vi "Dymin_v5.vi"() -> ()   [LabVIEW 2016]
doc: "This VI demonstrates how to use an external signal to control the execution rate of a while loop."
uses:
  <vilib>/Platform/TimedLoop/XDataNode/wakeup.ctl
  <vilib>/Platform/TimedLoop/XDataNode/XDNodeRunTimeDep.lvlib
  <vilib>/Platform/TimedLoop/XDataNode/nitl_modes.ctl
  <vilib>/Platform/TimedLoop/XDataNode/timing_clust.ctl
  <vilib>/Platform/TimedLoop/XDataNode/XDataNode.xnode
  <vilib>/eio/EIONode/EIONode.xnode
  <vilib>/rvi/eio/common/nirviEmuTemplateMethod_errors.vi
  <vilib>/rvi/DataTransferAndStorage/Container/XNode/niFpgaContainer.xnode
  <vilib>/rvi/FIFO/Fifo_Resource/niFpgaFifoEmulationRefIn.vi
panel:
  out "Index":i32
  out "Dymin Step":i32
  out "Counts":i32
  out "Last Index":i32
  out "Last Counts":i32
  in  "Time (#80MHz periods)":i32[](array[numeric])=[32, 32, 32, 32]
  in  "Threshold (counts)":i32[](array[numeric])=[0, 0, 0, 0]
  in  "AOM Volts (V)":i32[](array[numeric])=[0, 82, 164, 246]
  # "12 bit ADC volts"
  # ".1=82\n.2=164\n.3=246"
  # "16=200ns\n32=400ns"
  # "0 value means the step before it was the last step"
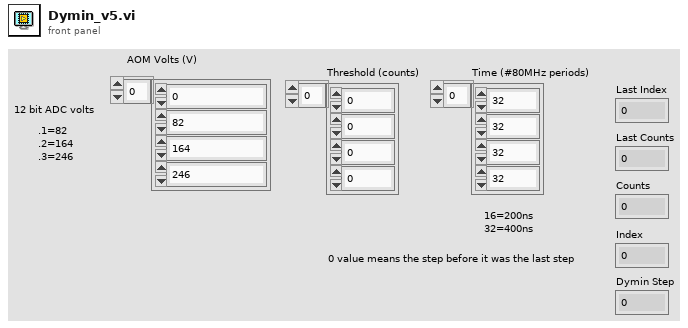
[diagram p1: front panel]
types:
  T1 = typedef "XDNodeRunTimeDep.lvlib/timing_clust.ctl" = cluster{"Expected End [f-1]":u64, "Actual End [f-1]":u64, "Finished Late? [f-1]":bool, "Expected End [i-1]":u64, "Actual End [i-1]":u64, "Finished Late? [i-1]":bool, "Expected Start [i]":u64, "Actual Start [i]":u64, "Expected Start [f]":u64, "Actual Start [f]":u64, "Source Name":string, "Structure Name":string, "Period":i64, "Deadline":i64, "Offset":i64, "Start":i64, "Priority":i32, "Timeout":i32, "Mode":T2, "Wakeup Reason":T3, "Error":errorcluster, "Source Type":string, "Secondary Source Type":string, "Global End Time":u64, "Global Start Time":u64, "Frame Duration":u64, "Iteration Duration":u64, "Assigned CPU":i32, "I/O Scan Engine Mode":u32}
  T2 = typedef "XDNodeRunTimeDep.lvlib/nitl_modes.ctl" = enum32{"No Change", "Process missed periods, maintain original phase", "Discard missed periods, maintain original phase", "Process missed periods, ignore original phase", "Discard missed periods, ignore original phase"}
  T3 = typedef "XDNodeRunTimeDep.lvlib/wakeup.ctl" = enum32{"Normal", "Aborted", "Asynchronous wakeup", "Timing source error", "Timed loop error", "Timeout"}
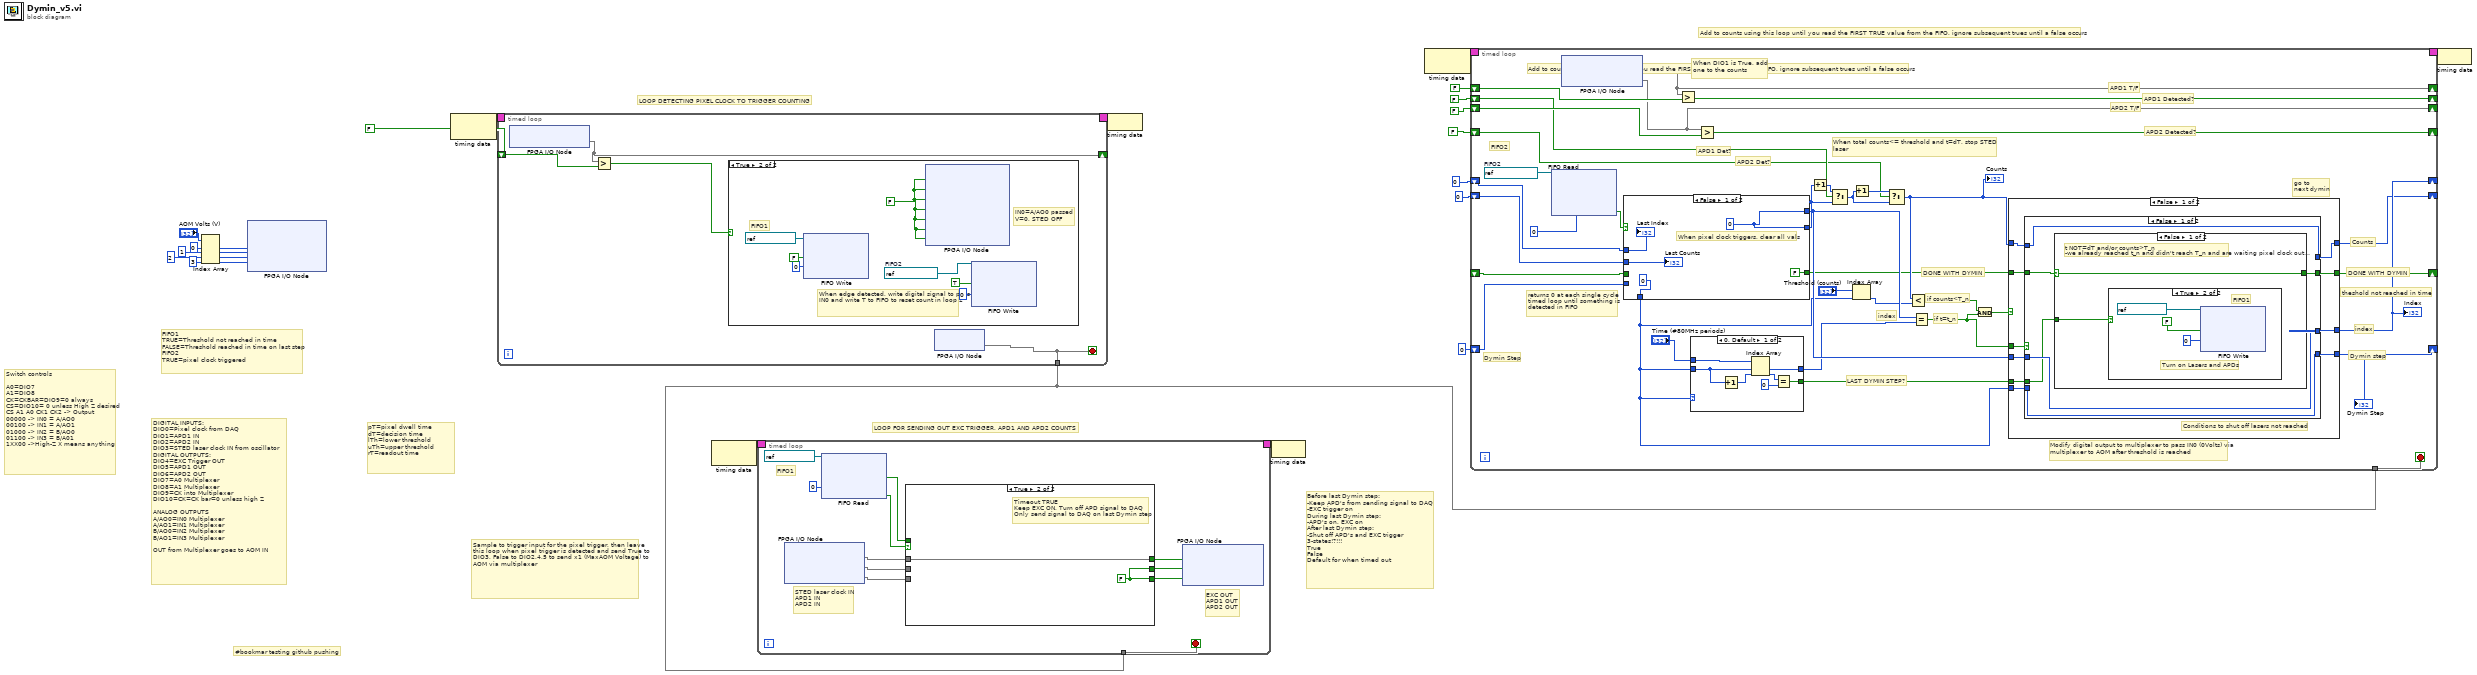
[diagram p0: block diagram]
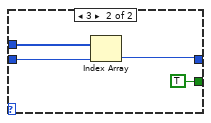
[diagram p2: hidden frame]
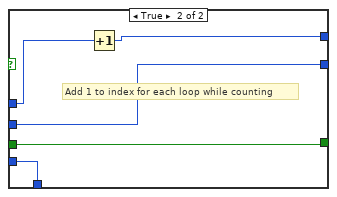
[diagram p3: hidden frame]
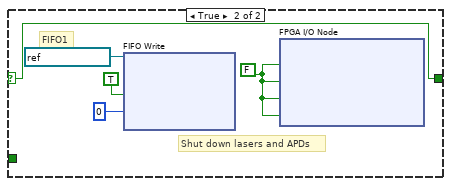
[diagram p5: hidden frame]
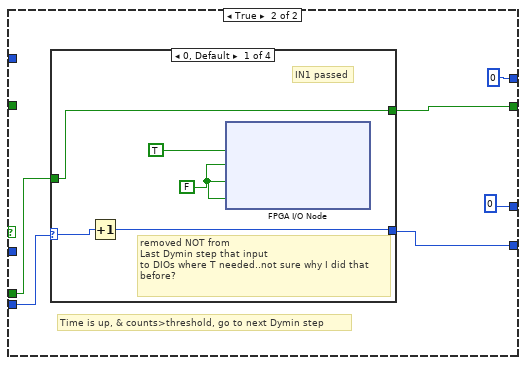
[diagram p6: hidden frame]
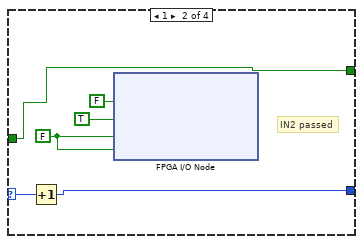
[diagram p7: hidden frame]
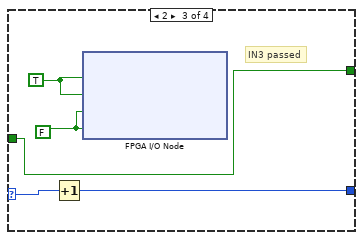
[diagram p8: hidden frame]
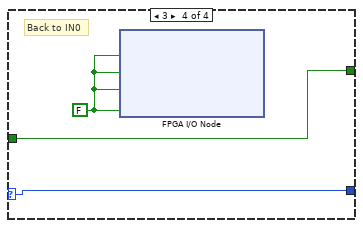
[diagram p9: hidden frame]
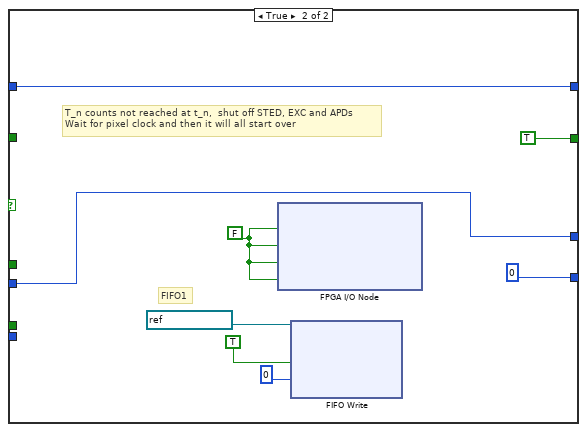
[diagram p10: hidden frame]
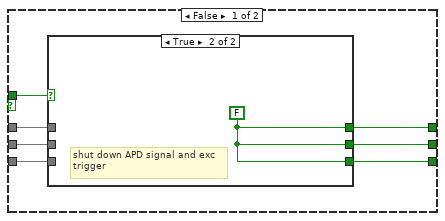
[diagram p11: hidden frame]
diagram:
  # "#bookmar testing github pushing"
  # "Switch controls\n\nA0=DIO7\nA1=DIO8\nCK=CKBAR=DIO9=0 always\nCS=DIO10= 0 unless High Z desired\nCS A1 A0 CK1 CK2 -> Output\n00000 -> IN0 = A/AO0\n00100 -> IN1 = A/AO1\n01000 -> IN2 = B/AO0\n01100 -> IN3 = B/A01\n1XX00 ->High-Z X means anything"
  # "FIFO1\nTRUE=Threshold not reached in time\nFALSE=Threshold reached in time on last step\nFIFO2\nTRUE=pixel clock triggered"
  # "DIGITAL INPUTS:\nDIO0=Pixel clock from DAQ\nDIO1=APD1 IN \nDIO2=APD2 IN\nDIO3=STED laser clock IN from oscillator\nDIGITAL OUTPUTS:\nDIO4=EXC Trigger OUT\nDIO5=APD1 OUT\nDIO6=APD2 OUT\nDIO7=A0 Multiplexer\nDIO8=A1 Multiplexer\nDIO9=CK into Multiplexer\nDIO10=CK=CK bar=0 unless high Z\n\nANALOG OUTPUTS\nA/AO0=IN0 Multiplexer\nA/AO1=IN1 Multiplexer\nB/AO0=IN2 Multiplexer\nB/AO1=IN3 Multiplexer\n\nOUT from Multiplexer goes to AOM IN"
  # "Before last Dymin step:\n-Keep APD's from sending signal to DAQ\n-EXC trigger on\nDuring last Dymin step:\n-APD's on, EXC on\nAfter last Dymin step:\n-Shut off APD's and EXC trigger\n3-states!?!!!\nTrue\nFalse\nDefault for when timed out"
  # "Add to counts using this loop until you read the FIRST TRUE value from the FIFO, ignore subsequent trues until a false occurs"
  # "LOOP FOR SENDING OUT EXC TRIGGER, APD1 AND APD2 COUNTS"
  # "LOOP DETECTING PIXEL CLOCK TO TRIGGER COUNTING"
  # "Add to counts using this loop until you read the FIRST TRUE value from the FIFO, ignore subsequent trues until a false occurs"
  # "Sample to trigger input for the pixel trigger, then leave this loop when pixel trigger is detected and send True to DIO3, False to DIO2,4,5 to send x1 (MaxAOM Voltage) to AOM via multiplexer"
  # "pT=pixel dwell time\ndT=decision time\nlTh=lower threshold\nuTh=upper threshold\nrT=readout time"
  n1 = Index Array(array="AOM Volts (V)", index #1=0 ("index"), index #2=1 ("index"), index #3=2 ("index"), index #4=3 ("index")) -> (element #1=w1:i32, element #2=w4:i32, element #3=w3:i32, element #4=w2:i32)
  n2 = xnode "FPGA I/O Node"("ConnectorA/AO0"=w1, "ConnectorA/AO1"=w4, "ConnectorB/AO0"=w3, "ConnectorB/AO1"=w2) -> ()  [unwired: 4 in, 4 out]
  n3 = node-c288() -> (w24:T1)  [unwired: 1 in]
  n4 = timed-loop {
    timing: w24 -> [_]
    timing-out: [_] -> w23
    shift-right: [w27] -> _
    shift-left: FALSE -> [w28]
    tunnel: [w25] -> w10
    stop <- w25 stop-if-true
    n5 = xnode "FPGA I/O Node"() -> ("ConnectorA/DIO0"=w27)  [unwired: 1 in, 1 out]
    n6 = Greater?(x=w27, y=w28) -> (0:w26:bool)
    n7 = case shown="True" w26 {
      frame False {
      }
      frame True {
        w29 = FALSE ("ConnectorA/DIO4")
        w35 = refnum<k21> "A.DO1 DMA"  # FIFO2
        # "FIFO1"
        # "When edge detected, write digital signal to pass IN0 and write T to FIFO to reset count in loop 2"
        # "IN0=A/AO0 passed\nV=0, STED OFF"
        n8 = xnode ("FIFO Write")("Element"=FALSE, "Timeout"=0, "FIFO In"=refnum<k21> "A.DI0 DMA") -> ()  [unwired: 2 out]
        n9 = xnode "FPGA I/O Node"("ConnectorA/DIO4"=w29, "ConnectorA/DIO5"=w29, "ConnectorA/DIO6"=w29, "ConnectorA/DIO7"=w29, "ConnectorA/DIO8"=w29, "ConnectorA/DIO9"=w29, "ConnectorA/DIO10"=w29) -> ()  [unwired: 7 in, 7 out]
        n10 = xnode ("FIFO Write")("Element"=TRUE, "Timeout"=0, "FIFO In"=w35) -> ()  [unwired: 2 out]
      }
    }
    n11 = xnode "FPGA I/O Node"() -> ("Button0"=w25)  [unwired: 1 in, 1 out]
  }
  n12 = node-c288() -> (w21:T1)  [unwired: 1 in]
  n13 = timed-loop {
    timing: w21 -> [_]
    timing-out: [_] -> w20
    tunnel: w10 -> [w38]
    stop <- w38 stop-if-true
    # "EXC OUT\nAPD1 OUT\nAPD2 OUT"
    # "FIFO1"
    # "STED laser clock IN\nAPD1 IN\nAPD2 IN"
    n14 = xnode "FPGA I/O Node"() -> ("ConnectorA/DIO3"=w46, "ConnectorA/DIO1"=w43, "ConnectorA/DIO2"=w42)  [unwired: 3 in, 3 out]
    n15 = xnode ("FIFO Read")("Timeout"=0, "FIFO In"=refnum<k21> "A.DI0 DMA") -> ("Element"=w45:bool, "Timed Out?"=w39:bool)  [unwired: 1 out]
    n16 = case shown="True" w39 {
      tunnel: w46 -> [w55 w61]
      tunnel: w45 -> [w54 _]
      tunnel: [w53 w61] -> w44
      tunnel: w43 -> [w52 _]
      tunnel: w42 -> [w51 _]
      tunnel: [w50 w60] -> w41
      tunnel: [w49 w60] -> w40
      frame False {
        n17 = case shown="True" w54 {
          tunnel: w55 -> [w58 _]
          tunnel: [w58 w59] -> w53
          tunnel: w52 -> [w57 _]
          tunnel: w51 -> [w56 _]
          tunnel: [w57 w59] -> w50
          tunnel: [w56 w59] -> w49
          frame False {
            # "Sends Exc Trig out, APD1 and APD2 out using FPGA"
          }
          frame True {
            w59 = FALSE ("ConnectorA/DIO3")
            # "shut down APD signal and exc trigger"
          }
        }
      }
      frame True {
        w60 = FALSE
        # "Timeout TRUE\nKeep EXC ON, Turn off APD signal to DAQ\nOnly send signal to DAQ on last Dymin step"
      }
    }
    n18 = xnode "FPGA I/O Node"("ConnectorA/DIO4"=w44, "ConnectorA/DIO5"=w41, "ConnectorA/DIO6"=w40) -> ()  [unwired: 3 in, 3 out]
  }
  n19 = node-c288(w23) -> ()
  n20 = node-c288(w20) -> ()
  n21 = node-c288() -> (w19:T1)  [unwired: 1 in]
  n22 = timed-loop {
    timing: w19 -> [_]
    timing-out: [_] -> w18
    shift-right: [w97] -> _
    shift-left: FALSE -> [w99]
    shift-right: [w91] -> _
    shift-left: FALSE -> [w86]
    shift-right: [w80] -> _
    shift-left: 0 -> [w94]
    shift-right: [w75] -> _
    shift-left: FALSE -> [w87]
    shift-right: [w92] -> _
    shift-left: FALSE -> [w90]
    shift-right: [w76] -> _
    shift-left: 0 -> [w88]
    shift-right: [w82] -> _
    shift-left: 0 -> [w66]
    shift-right: [w70] -> _
    shift-left: _ -> [w68]
    tunnel: w10 -> [w64]
    stop <- w64 stop-if-true
    w79 = refnum<k21> "A.DO1 DMA"  # FIFO2
    # "DONE WITH DYMIN"
    # "go to\nnext dymin"
    # "DONE WITH DYMIN"
    # "LAST DYMIN STEP?"
    # "theshold not reached in time"
    # "Dymin Step"
    # "Dymin step"
    # "FIFO2"
    # "if counts<T_n"
    # "if t=t_n"
    # "returns 0 at each single cycle timed loop until something is detected in FIFO"
    # "Modify digital output to multiplexer to pass IN0 (0Volts) via multiplexer to AOM after threshold is reached"
    # "When total counts<= threshold and t=dT, stop STED laser"
    # "index"
    # "APD1 Det?"
    # "APD2 Det?"
    # "APD2 Detected?"
    # "APD2 T/F"
    # "APD1 Detected?"
    # "APD1 T/F"
    # "index"
    # "Counts"
    # "When DIO1 is True, add one to the counts"
    n23 = xnode ("FIFO Read")("Timeout"=0, "FIFO In"=w79) -> ("Timed Out?"=w93:bool)  [unwired: 2 out]
    n24 = xnode "FPGA I/O Node"() -> ("ConnectorA/DIO1"=w97, "ConnectorA/DIO2"=w92)  [unwired: 2 in, 2 out]
    n25 = case shown="False" w93 {
      tunnel: [w114 w118] -> w95
      tunnel: [w114 w119] -> w81
      tunnel: w94 -> [w115 w120]
      tunnel: w88 -> [w113 w118]
      tunnel: w68 -> [_ w117]
      tunnel: [FALSE w117] -> w67
      tunnel: w66 -> [_ w116]
      tunnel: [0 w116] -> w65
      frame False {
        w114 = 0
        # "When pixel clock triggers, clear all vals"
        "Last Index" <- w115
        "Last Counts" <- w113
      }
      frame True {
        # "Add 1 to index for each loop while counting"
        n26 = Increment(x=w120) -> (x+1=w119:i32)
      }
    }
    n27 = Greater?(x=w97, y=w99) -> (0:w75:bool)
    n28 = case shown="0, Default" w65 {
      tunnel: [w106 w108] -> w74
      tunnel: w65 -> [w104 w109]
      tunnel: [w101 TRUE] -> w72
      tunnel: "Time (#80MHz periods)" -> [w100 w110]
      frame 0, Default {
        n29 = Increment(x=w104) -> (x+1=w105:i32)
        n30 = Index Array(array=w100, index #1=w104, index #2=w105) -> (element #1=w106:i32, element #2=w103:i32)
        n31 = Equal?(x=w103, y=0) -> (x = y?=w101:bool)
      }
      frame 3 {
        n32 = Index Array(array=w110, index=w109) -> (element=w108:i32)
      }
    }
    n33 = Greater?(x=w92, y=w90) -> (0:w91:bool)
    n34 = Increment(x=w95) -> (x+1=w98:i32)
    n35 = Select(t=w98, s=w87, f=w95) -> (s? t:f=w83:i32)
    n36 = Index Array(array="Threshold (counts)", index=w65) -> (element=w73:i32)
    n37 = Increment(x=w83) -> (x+1=w89:i32)
    n38 = Select(t=w89, s=w86, f=w83) -> (s? t:f=w77:i32)
    "Counts" <- w77
    n39 = Less?(x=w77, y=w73) -> (x < y?=w85:bool)
    n40 = Equal?(x=w81, y=w74) -> (x = y?=w71:bool)
    n41 = And(x=w85, y=w71) -> (x .and. y?=w84:bool)
    n42 = case shown="False" w84 {
      tunnel: w65 -> [w130 _]
      tunnel: [w129 0] -> w82
      tunnel: w81 -> [w128 w176]
      tunnel: [w127 w176] -> w80
      tunnel: w77 -> [w125 w174]
      tunnel: [w126 w174] -> w76
      tunnel: w72 -> [w124 _]
      tunnel: w71 -> [w123 _]
      tunnel: [w122 TRUE] -> w70
      tunnel: w67 -> [w121 _]
      frame False {
        # "Conditions to shut off lasers not reached"
        n43 = case shown="False" w123 {
          tunnel: w130 -> [w136 w150]
          tunnel: [w136 w149] -> w129
          tunnel: w128 -> [w135 _]
          tunnel: [w135 0] -> w127
          tunnel: [w134 0] -> w126
          tunnel: w125 -> [w134 _]
          tunnel: w124 -> [w131 w148]
          tunnel: [w133 w147] -> w122
          tunnel: w121 -> [w132 _]
          frame False {
            # "t NOT=dT and/or counts>T_n\n-we already reached t_n and didn't reach T_n and are waiting pixel clock out\n-we haven't reached t_n and are waiting\n-"
            n44 = case shown="False" w132 {
              selector: w132 -> [w138 w142]
              tunnel: [w138 w142] -> w133
              tunnel: w131 -> [w137 _]
              frame False {
                n45 = case shown="True" w137 {
                  frame False {
                  }
                  frame True {
                    # "Turn on Lasers and APDs"
                    # "FIFO1"
                    n46 = xnode ("FIFO Write")("Element"=FALSE, "Timeout"=0, "FIFO In"=refnum<k21> "A.DI0 DMA") -> ()  [unwired: 2 out]
                  }
                }
              }
              frame True {
                w143 = FALSE
                # "Shut down lasers and APDs"
                # "FIFO1"
                n47 = xnode ("FIFO Write")("Element"=TRUE, "Timeout"=0, "FIFO In"=refnum<k21> "A.DI0 DMA") -> ()  [unwired: 2 out]
                n48 = xnode "FPGA I/O Node"("ConnectorA/DIO7"=w143, "ConnectorA/DIO8"=w143, "ConnectorA/DIO9"=w143, "ConnectorA/DIO10"=w143) -> ()  [unwired: 4 in, 4 out]
              }
            }
          }
          frame True {
            # "Time is up, & counts>threshold, go to next Dymin step"
            n49 = case shown="0, Default" w150 {
              selector: w150 -> [w157 w163 w168 w169]
              tunnel: [w156 w162 w167 w169] -> w149
              tunnel: w148 -> [w154 w160 w166 w170]
              tunnel: [w154 w160 w166 w170] -> w147
              frame 0, Default {
                w155 = FALSE ("ConnectorA/DIO4")
                # "removed NOT from\nLast Dymin step that input\nto DIOs where T needed..not sure why I did that\nbefore?"
                # "IN1 passed"
                n50 = Increment(x=w157) -> (x+1=w156:i32)
                n51 = xnode "FPGA I/O Node"("ConnectorA/DIO7"=TRUE, "ConnectorA/DIO8"=w155, "ConnectorA/DIO9"=w155, "ConnectorA/DIO10"=w155) -> ()  [unwired: 4 in, 4 out]
              }
              frame 1 {
                w161 = FALSE ("ConnectorA/DIO4")
                # "IN2 passed"
                n52 = Increment(x=w163) -> (x+1=w162:i32)
                n53 = xnode "FPGA I/O Node"("ConnectorA/DIO7"=FALSE, "ConnectorA/DIO8"=TRUE, "ConnectorA/DIO9"=w161, "ConnectorA/DIO10"=w161) -> ()  [unwired: 4 in, 4 out]
              }
              frame 2 {
                w165 = TRUE ("ConnectorA/DIO7")
                w164 = FALSE ("ConnectorA/DIO4")
                # "IN3 passed"
                n54 = Increment(x=w168) -> (x+1=w167:i32)
                n55 = xnode "FPGA I/O Node"("ConnectorA/DIO7"=w165, "ConnectorA/DIO8"=w165, "ConnectorA/DIO9"=w164, "ConnectorA/DIO10"=w164) -> ()  [unwired: 4 in, 4 out]
              }
              frame 3 {
                w171 = FALSE ("ConnectorA/DIO4")
                # "Back to IN0"
                n56 = xnode "FPGA I/O Node"("ConnectorA/DIO7"=w171, "ConnectorA/DIO8"=w171, "ConnectorA/DIO9"=w171, "ConnectorA/DIO10"=w171) -> ()  [unwired: 4 in, 4 out]
              }
            }
          }
        }
      }
      frame True {
        w179 = FALSE
        # "T_n counts not reached at t_n,  shut off STED, EXC and APDs\nWait for pixel clock and then it will all start over"
        # "FIFO1"
        n57 = xnode "FPGA I/O Node"("ConnectorA/DIO7"=w179, "ConnectorA/DIO8"=w179, "ConnectorA/DIO9"=w179, "ConnectorA/DIO10"=w179) -> ()  [unwired: 4 in, 4 out]
        n58 = xnode ("FIFO Write")("Element"=TRUE, "Timeout"=0, "FIFO In"=refnum<k21> "A.DI0 DMA") -> ()  [unwired: 2 out]
      }
    }
    "Dymin Step" <- w82
    "Index" <- w80
  }
  n59 = node-c288(w18) -> ()
